vi "GetStartTime.vi"   [LabVIEW 2010]
uses:
  5.0-Global.vi
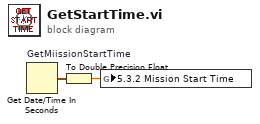
[diagram p0: block diagram]
diagram:
  n1 = Get Date/Time In Seconds "GetMiissionStartTime"() -> (seconds since 1Jan1904=w1:timestamp)
  n2 = To Double Precision Float(number=w1) -> (double precision float=w2:dbl)
  n3 = global write "5.0-Global.vi" "5.3.2 Mission Start Time"(w2) -> ()
